vi "Resubscribe.vi"(8 "error in (no error)":errorcluster, 11 "STOMP in":refnum<class "STOMP.lvclass">) -> (0 "error out":errorcluster, 3 "STOMP out":refnum<class "STOMP.lvclass">)   [LabVIEW 2017, in "LabVIEW STOMP.lvlib" / "STOMP.lvclass"]
uses:
  STOMP.lvclass
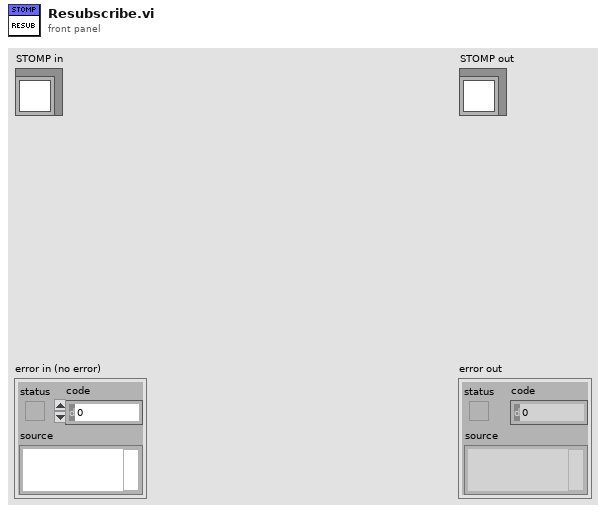
[diagram p1: front panel]
types:
  T1 = typedef "STOMP Connection Manager.lvclass/ObjectAttributes.ctl" = cluster{"address":string, "port":u16, "ConnectionRef":refnum<k5>, "messageQueue":refnum<queue>, "receiptQueue":refnum<queue>, "errorQueue":refnum<queue>, "sendQueue":refnum<queue>, "currentReceiptNumber":u64, "currentSubscriptionId":u64, "closeConnection":bool, "activeSubscriptions":T2[]}
  T2 = typedef "LabVIEW STOMP.lvlib/STOMP.lvclass/Type_ActiveSubscription.ctl" = cluster{"id":u64, "receipt":bool, "Destination":string, "ack":T3, "headers":T4[]}
  T3 = typedef "LabVIEW STOMP.lvlib/STOMP.lvclass/Type_AckHeader.ctl" = enum16{"auto", "client", "client-individual"}
  T4 = typedef "LabVIEW STOMP.lvlib/STOMP.lvclass/Type_FrameHeader.ctl" = cluster{"Header":string, "Value":string}
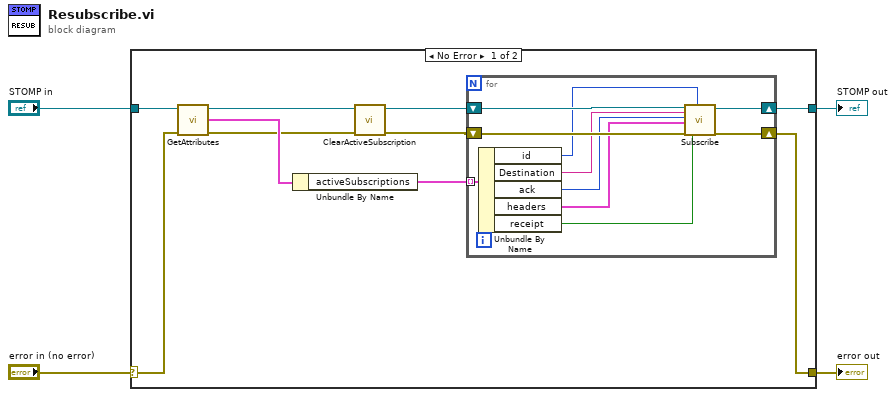
[diagram p0: block diagram]
diagram:
  n1 = case shown="No Error" "error in (no error)" {
    selector: "error in (no error)" -> [w13 w26]
    tunnel: [w9 w26] -> w3
    tunnel: [w11 w25] -> w1
    tunnel: "STOMP in" -> [w14 w25]
    frame No Error {
      n2 = call-dynamic "GetAttributes.vi"("error in (no error)"=w13, "STOMP in"=w14) -> ("error out"=w7:errorcluster, "attributes"=w12:T1, "STOMP out"=w8:refnum<class "STOMP.lvclass">)  [unwired: 7 in]
      n3 = Unbundle By Name(w12) -> ("activeSubscriptions"=w10:T2[])
      n4 = call-dynamic "ClearActiveSubscription.vi"("error in (no error)"=w7, "STOMP in"=w8) -> ("error out"=w6:errorcluster, "STOMP out"=w5:refnum<class "STOMP.lvclass">)  [unwired: 8 in]
      n5 = for {
        shift-right: [w20] -> w11
        shift-left: w5 -> [w23]
        tunnel: w10 -> [w24] mode=indexing
        shift-right: [w21] -> w9
        shift-left: w6 -> [w22]
        n6 = Unbundle By Name(w24) -> ("id"=w15:u64, "Destination"=w19:string, "ack"=w18:T3, "headers"=w17:T4[], "receipt"=w16:bool)
        n7 = call-dynamic "Subscribe.vi"("STOMP in"=w23, "Destination"=w19, "ack"=w18, "headers"=w17, "error in (no error)"=w22, "Receipt?"=w16, "ForceId"=w15) -> ("STOMP out"=w20:refnum<class "STOMP.lvclass">, "error out"=w21:errorcluster)  [unwired: 10 in, 1 out]
      }
    }
    frame Error {
    }
  }
  "error out" <- w3
  "STOMP out" <- w1
